vi "Supercell Structure into a Box 2014-11-11.vi"(8 "Keep old lattice vectors?":bool, 9 "Center Subcrystal":bool, 10 "Draw Box":T2, 11 "Subcrystal":T1={"Structure Name"="Gamm8 Subcrystal", "Lattice vector a"=[2.3379684769090283, 4.050155798593294, -3.073453095936429e-05], "Lattice vector b"=[0.0, 2.7000749366574968, 3.8175198422845327], "Lattice vector c"=[4.675927601962877, 0.0, 0.0], "Atoms Array"=[{"Atom Name"="Cd", "Positions (Direct)"=[[0.0, 2.2797955771e-06, 0.2499966378910753]], "Positions (Cartesian)"=[[0.0, -3.2294507389786483e-06, 2.863111017657439]]}, {"Atom Name"="Te", "Positions (Direct)"=[[0.0, -2.2797955771e-06, 3.3621089247e-06]], "Positions (Cartesian)"=[[0.0, -1.5237858666867705e-05, -2.8630725126350507]]}], "# of atoms"=2} {"Atoms Array"."Positions (Cartesian)" format="%#_4f"; "Atoms Array"."Positions (Direct)" format="%#_4f"}) -> (2 "Supercells Filled":dbl[][](array[numeric]), 3 "Expanded cubic Structure":T1={"Structure Name"="Gamm8 Subcrystal", "Lattice vector a"=[2.3379684769090283, 4.050155798593294, -3.073453095936429e-05], "Lattice vector b"=[0.0, 2.7000749366574968, 3.8175198422845327], "Lattice vector c"=[4.675927601962877, 0.0, 0.0], "Atoms Array"=[{"Atom Name"="Cd", "Positions (Direct)"=[[0.0, 2.2797955771e-06, 0.2499966378910753]], "Positions (Cartesian)"=[[0.0, -3.2294507389786483e-06, 2.863111017657439]]}, {"Atom Name"="Te", "Positions (Direct)"=[[0.0, -2.2797955771e-06, 3.3621089247e-06]], "Positions (Cartesian)"=[[0.0, -1.5237858666867705e-05, -2.8630725126350507]]}], "# of atoms"=2} {"Atoms Array"."Positions (Cartesian)" format="%#_4f"; "Atoms Array"."Positions (Direct)" format="%#_4f"})   [LabVIEW 2010]
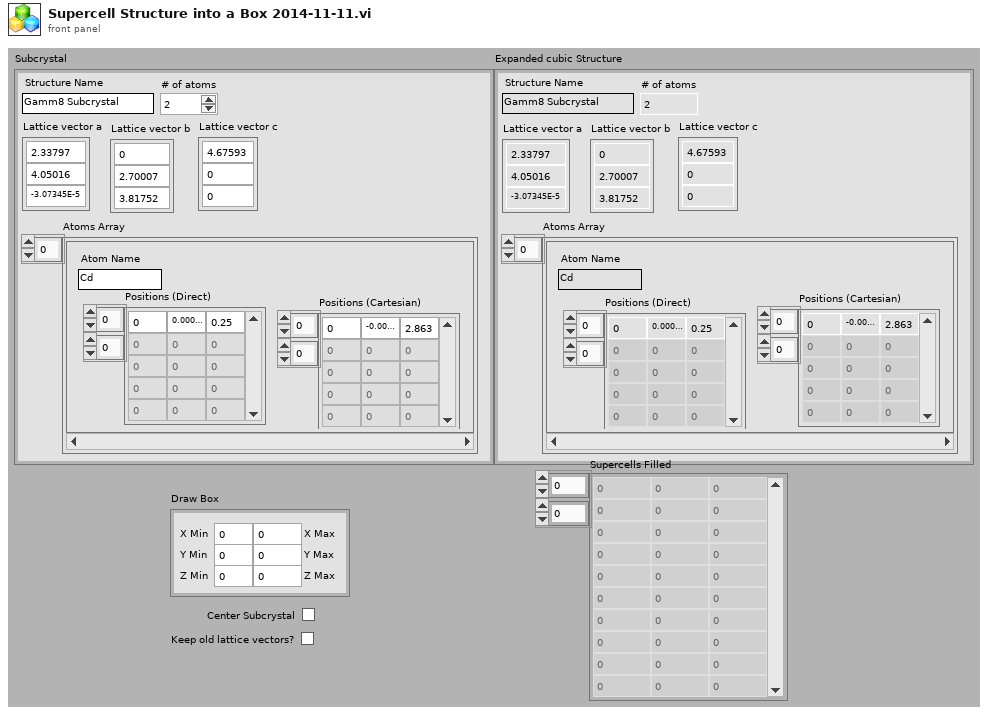
[diagram p1: front panel]
types:
  T1 = cluster{"Structure Name":string, "Lattice vector a":dbl[], "Lattice vector b":dbl[], "Lattice vector c":dbl[], "Atoms Array":cluster{"Atom Name":string, "Positions (Direct)":dbl[][], "Positions (Cartesian)":dbl[][]}[], "# of atoms":i32}
  T2 = cluster{"X Min":dbl, "X Max":dbl, "Y Min":dbl, "Y Max":dbl, "Z Min":dbl, "Z Max":dbl}
  T3 = cluster{"Atom Name":string, "Positions (Direct)":dbl[][], "Positions (Cartesian)":dbl[][]}[]
  T4 = cluster{"Atom Name":string, "Positions (Direct)":dbl[][], "Positions (Cartesian)":dbl[][]}
  T5 = cluster{"Atom Name":string, "Positions (Direct)":dbl[][], "Output Array":dbl[][]}
  T6 = cluster{string, "Lattice vector a":dbl[], "Lattice vector b":dbl[], "Lattice vector c":dbl[], cluster{"Atom Name":string, "Positions (Direct)":dbl[][], "Output Array":dbl[][]}[], i32}
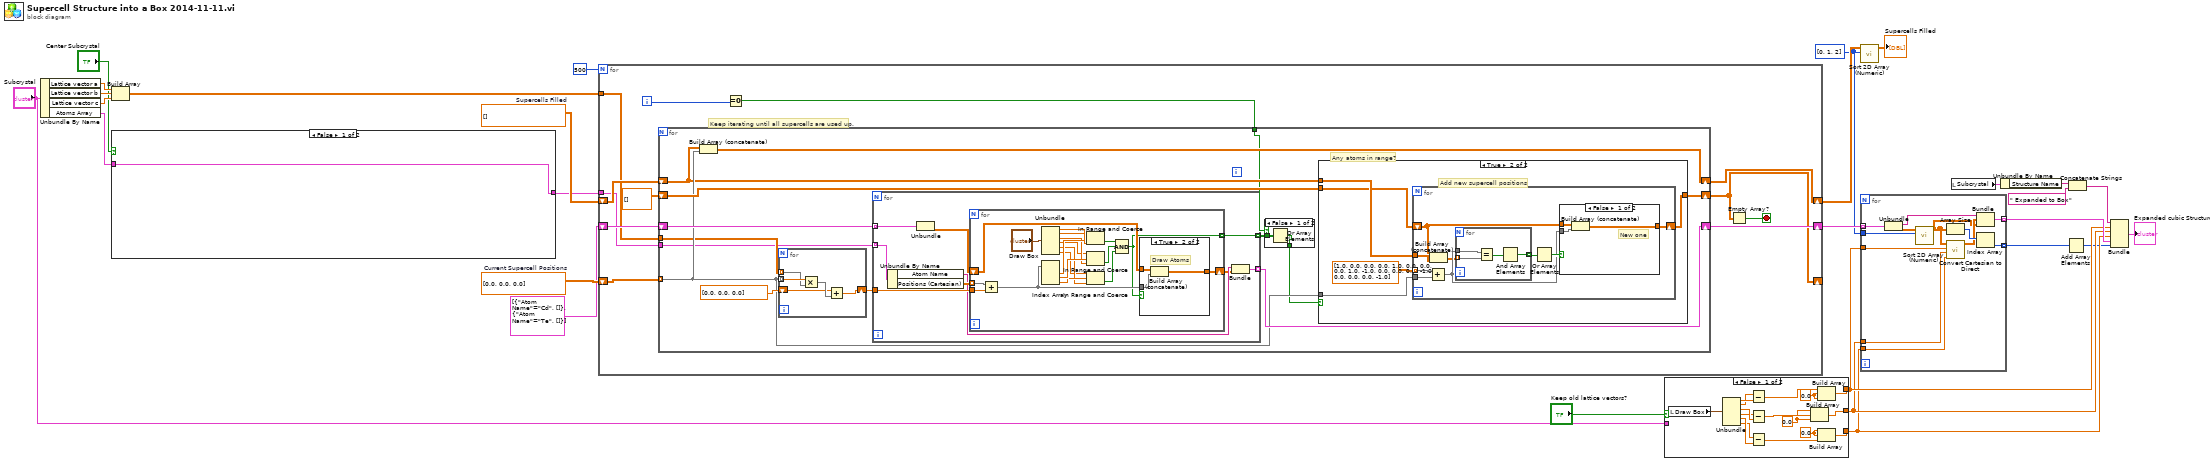
[diagram p0: block diagram]
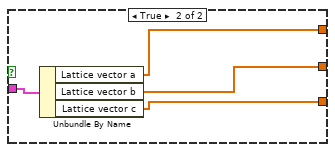
[diagram p2: hidden frame]
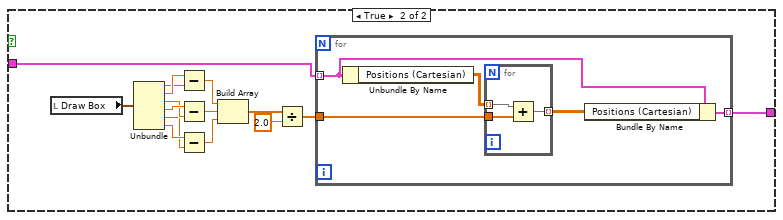
[diagram p7: hidden frame]
diagram:
  w14 = i32[] [0, 1, 2] ("Sort by Cols")
  w26 = dbl[][] []  # Supercells Filled
  w28 = dbl[][] [[0.0, 0.0, 0.0]]  # Current Supercell Positions
  n1 = Unbundle By Name("Subcrystal") -> ("Lattice vector a"=w24:dbl[], "Lattice vector b"=w23:dbl[], "Lattice vector c"=w22:dbl[], "Atoms Array"=w25:T3)
  n2 = Build Array(w24, w23, w22) -> (w21:dbl[][])
  n3 = case shown="False" "Center Subcrystal" {
    tunnel: w25 -> [w29 w44]
    tunnel: [w29 w30] -> w20
    frame False {
    }
    frame True {
      n4 = local read "Draw Box"() -> (w43:T2)
      n5 = Unbundle(w43) -> ("X Min"=w41:dbl, "X Max"=w42:dbl, "Y Min"=w38:dbl, "Y Max"=w39:dbl, "Z Min"=w35:dbl, "Z Max"=w36:dbl)
      n6 = Subtract(x=w42, y=w41) -> (x-y=w40:dbl)
      n7 = Subtract(x=w39, y=w38) -> (x-y=w37:dbl)
      n8 = Subtract(x=w36, y=w35) -> (x-y=w34:dbl)
      n9 = Build Array(w40, w37, w34) -> (w33:dbl[])
      n10 = Divide(x=w33, y=2.0) -> (x/y=w31:dbl[])
      n11 = for {
        tunnel: w44 -> [w47] mode=indexing
        tunnel: w31 -> [w48]
        tunnel: [w45] -> w30 mode=indexing
        n12 = Unbundle By Name(w47) -> ("Positions (Cartesian)"=w49:dbl[][])
        n13 = for {
          tunnel: w49 -> [w52] mode=indexing
          tunnel: w48 -> [w51]
          tunnel: [w50] -> w46 mode=indexing
          n14 = Add(x=w52, y=w51) -> (x+y=w50:dbl[])
        }
        n15 = Bundle By Name(cluster=w47, "Positions (Cartesian)"=w46) -> (w45:T4)
      }
    }
  }
  n16 = for {
    N: 500 -> [_]
    shift-right: [w56] -> _
    shift-left: w28 -> [w64]
    shift-right: [w62] -> w15
    shift-left: cluster{"Atom Name":string, dbl[][]}[] [{"Atom Name"="Cd", []}, {"Atom Name"="Te", []}] -> [w61]
    shift-right: [w59] -> w18
    shift-left: w26 -> [w60]
    tunnel: w21 -> [w58]
    tunnel: w20 -> [w57]
    i -> [w54]
    stop <- w55 stop-if-true
    # "Keep iterating until all supercells are used up."
    n17 = Equal To 0?(x=w54) -> (x = 0?=w53:bool)
    n18 = for {
      shift-right: [w73] -> w56
      shift-left: dbl[][] [] ("Supercell Positions") -> [w76]
      tunnel: w64 -> [w72] mode=indexing
      shift-right: [w75] -> w62
      shift-left: w61 -> [w74]
      shift-right: [w68] -> w59
      shift-left: w60 -> [w71]
      tunnel: w58 -> [w70]
      tunnel: w57 -> [w69]
      tunnel: w53 -> [w65]
      # "Any atoms in range?"
      n19 = Build Array (concatenate)(w71, w72) -> (w68:dbl[][])
      n20 = for {
        tunnel: w72 -> [w109] mode=indexing
        shift-right: [w107] -> w77
        shift-left: dbl[] [0.0, 0.0, 0.0] -> [w106]
        tunnel: w70 -> [w105] mode=indexing
        n21 = Multiply(x=w109, y=w105) -> (x*y=w108:dbl[])
        n22 = Add(x=w106, y=w108) -> (x+y=w107:dbl[])
      }
      n23 = for {
        tunnel: w69 -> [w116] mode=indexing
        tunnel: w77 -> [w117]
        tunnel: [w115] -> w67 mode=indexing
        tunnel: w74 -> [w111] mode=indexing
        tunnel: [w112] -> w75 mode=indexing
        n24 = Unbundle By Name(w116) -> ("Atom Name"=w114:string, "Positions (Cartesian)"=w118:dbl[][])
        n25 = Unbundle(w111) -> (w110:dbl[][])  [unwired: 1 out]
        n26 = for {
          tunnel: w118 -> [w137] mode=indexing
          tunnel: w117 -> [w136]
          shift-right: [w121] -> w113
          shift-left: w110 -> [w120]
          tunnel: [w119] -> w115 mode=indexing
          n27 = Add(x=w137, y=w136) -> (x+y=w122:dbl[])
          n28 = Unbundle("Draw Box") -> ("X Min"=w134:dbl, "X Max"=w133:dbl, "Y Min"=w129:dbl, "Y Max"=w128:dbl, "Z Min"=w127:dbl, "Z Max"=w126:dbl)
          n29 = Index Array(array=w122) -> (element #1=w132:dbl, element #2=w131:dbl, element #3=w130:dbl)  [unwired: 3 in]
          n30 = In Range and Coerce(upper limit=w133, x=w132, lower limit=w134) -> (In Range?=w125:bool)  [unwired: 1 out]
          n31 = In Range and Coerce(upper limit=w128, x=w131, lower limit=w129) -> (In Range?=w124:bool)  [unwired: 1 out]
          n32 = In Range and Coerce(upper limit=w126, x=w130, lower limit=w127) -> (In Range?=w123:bool)  [unwired: 1 out]
          n33 = Compound Arithmetic op=AND(w125, w124, w123) -> (w119:bool)
          n34 = case shown="True" w119 {
            tunnel: w122 -> [_ w141]
            tunnel: [w138 w140] -> w121
            tunnel: w120 -> [w138 w139]
            frame False {
              # "Not inside box"
            }
            frame True {
              # "Draw Atoms"
              n35 = Build Array (concatenate)(w139, w141) -> (w140:dbl[][])
            }
          }
        }
        n36 = Bundle("Atom Name"=w114, w113) -> (w112:cluster{"Atom Name":string, dbl[][]})  [unwired: 1 in]
      }
      n37 = case shown="False" w65 {
        selector: w65 -> [_ w81]
        tunnel: w67 -> [w80 _]
        tunnel: [w79 w81] -> w66
        frame False {
          n38 = Or Array Elements(Boolean array=w80) -> (logical OR=w79:bool)
        }
        frame True {
        }
      }
      n39 = case shown="True" w66 {
        tunnel: w72 -> [_ w87]
        tunnel: [w82 w83] -> w73
        tunnel: w76 -> [w82 w84]
        tunnel: w71 -> [_ w85]
        frame False {
          # "Don't sweat it"
        }
        frame True {
          # "Add new supercell positions"
          n40 = for {
            tunnel: w87 -> [w95]
            tunnel: dbl[][] [[1.0, 0.0, 0.0], [0.0, 1.0, 0.0], [0.0, 0.0, 1.0], [-1.0, 0.0, 0.0], [0.0, -1.0, 0.0], [0.0, 0.0, -1.0]] -> [w96] mode=indexing
            tunnel: w85 -> [w90]
            shift-right: [w94] -> w83
            shift-left: w84 -> [w89]
            n41 = Add(x=w96, y=w95) -> (x+y=w92:dbl[])
            n42 = Build Array (concatenate)(w90, w89) -> (w88:dbl[][])
            n43 = for {
              tunnel: w92 -> [w104]
              tunnel: w88 -> [w103] mode=indexing
              tunnel: [w101] -> w91 mode=indexing
              n44 = Equal?(x=w104, y=w103) -> (x = y?=w102:bool[])
              n45 = And Array Elements(Boolean array=w102) -> (logical AND=w101:bool)
            }
            n46 = Or Array Elements(Boolean array=w91) -> (logical OR=w93:bool)
            n47 = case shown="False" w93 {
              tunnel: w92 -> [w99 _]
              tunnel: [w98 w100] -> w94
              tunnel: w89 -> [w97 w100]
              frame False {
                # "New one"
                n48 = Build Array (concatenate)(w97, w99) -> (w98:dbl[][])
              }
              frame True {
                # "Already Did this one"
              }
            }
          }
        }
      }
    }
    n49 = Empty Array?(array=w56) -> (empty?=w55:bool)
  }
  n50 = case shown="False" "Keep old lattice vectors?" {
    tunnel: [w144 w160] -> w12
    tunnel: [w143 w159] -> w11
    tunnel: [w142 w158] -> w10
    tunnel: "Subcrystal" -> [_ w161]
    frame False {
      w146 = 0.0 ("element")
      w147 = 0.0 ("element")
      w150 = 0.0 ("element")
      n51 = local read "Draw Box"() -> (w151:T2)
      n52 = Unbundle(w151) -> ("X Min"=w153:dbl, "X Max"=w152:dbl, "Y Min"=w155:dbl, "Y Max"=w154:dbl, "Z Min"=w157:dbl, "Z Max"=w156:dbl)
      n53 = Subtract(x=w152, y=w153) -> (x-y=w149:dbl)
      n54 = Subtract(x=w154, y=w155) -> (x-y=w148:dbl)
      n55 = Subtract(x=w156, y=w157) -> (x-y=w145:dbl)
      n56 = Build Array(w147, w148, w147) -> (w143:dbl[])
      n57 = Build Array(w149, w150, w150) -> (w144:dbl[])
      n58 = Build Array(w146, w146, w145) -> (w142:dbl[])
    }
    frame True {
      n59 = Unbundle By Name(w161) -> ("Lattice vector a"=w160:dbl[], "Lattice vector b"=w159:dbl[], "Lattice vector c"=w158:dbl[])
    }
  }
  n60 = call "Sort 2D Array (Numeric).vi"("Sort by Cols"=w14, "Input Array"=w18) -> ("Output Array"=→"Supercells Filled":dbl[][])  [unwired: 9 in]
  n61 = for {
    tunnel: w15 -> [w173] mode=indexing
    tunnel: w14 -> [w171]
    tunnel: [w169] -> w13 mode=indexing
    tunnel: w12 -> [w168]
    tunnel: w11 -> [w167]
    tunnel: w10 -> [w166]
    tunnel: [w164] -> w5 mode=indexing
    n62 = Unbundle(w173) -> ("Atom Name"=w170:string, w172:dbl[][])
    n63 = call "Sort 2D Array (Numeric).vi"("Sort by Cols"=w171, "Input Array"=w172) -> ("Output Array"=w162:dbl[][])  [unwired: 9 in]
    n64 = Array Size(array=w162) -> (size(s)=w165:i32[])
    n65 = call "Convert Cartesian to Direct.vi"("Lattice vector c"=w166, "Lattice vector b"=w167, "Lattice vector a"=w168, "Positions (Cartesian)"=w162) -> ("Positions (Direct)"=w163:dbl[][])  [unwired: 7 in]
    n66 = Bundle("Atom Name"=w170, "Positions (Direct)"=w163, "Output Array"=w162) -> (w169:T5)  [unwired: 1 in]
    n67 = Index Array(array=w165) -> (element=w164:i32)  [unwired: 1 in]
  }
  n68 = local read "Subcrystal"() -> (w9:T1)
  n69 = Unbundle By Name(w9) -> ("Structure Name"=w8:string)
  n70 = Add Array Elements(numeric array=w5) -> (sum=w4:i32)
  n71 = Concatenate Strings(w8, " Expanded to Box" ("string")) -> (w6:string)
  n72 = Bundle(w6, "Lattice vector a"=w12, "Lattice vector b"=w11, "Lattice vector c"=w10, w13, w4) -> (→"Expanded cubic Structure":T6)  [unwired: 1 in]
